vi "Login.vi"(8 "error in (no error)":errorcluster, 11 "UI in":refnum<class "UI.lvclass">) -> (0 "error out":errorcluster, 3 "UI out":refnum<class "UI.lvclass">)   [LabVIEW 2018]
uses:
  User Interface/UI.lvclass
  controls/DataIn.ctl
  MatchDataClasses/MatchData/MatchData.lvclass
  controls/Tabuleiro.ctl
  controls/Table.ctl
  User Interface/UI.lvclass/UI.ctl
  controls/LoginStatus.ctl
  User Interface/getUIData.vi
  User Interface/setUIData.vi
  User Interface/setEmbeddedVI.vi
  <vilib>/Utility/file.llb/Read Delimited Spreadsheet (string).vi
  <vilib>/Utility/file.llb/Write Delimited Spreadsheet (string).vi
panel:
  out "DataOut":T1={"Quem Joga"="", "Tabuleiro"={"(0,0)"="", "(1,0)"="", "(0,1)"="", "(1,1)"="", "(2,0)"="", "(1,2)"="", "(2,2)"="", "(0,2)"="", "(2,1) "=""}, "GameOption"=enum."Multiplayer local", "Turno"=FALSE, "Player"="", "Player 1"="", "Player 2"="", "Dificuldade"=enum."Easy", "Table"=[], "Row"=0, "Aceitar Convite"=FALSE, "Inviter line"=0, "diretório"=path "", "Logout - panel close"=FALSE, "StartGame"=FALSE, "MatchData.lvclass"=refnum, "GameMode"=enum."Single Easy", "Level State"=FALSE}
  out "Table":string[][](table)
  in  "logout":bool
  in  "Login":bool
  in  "User Name":string
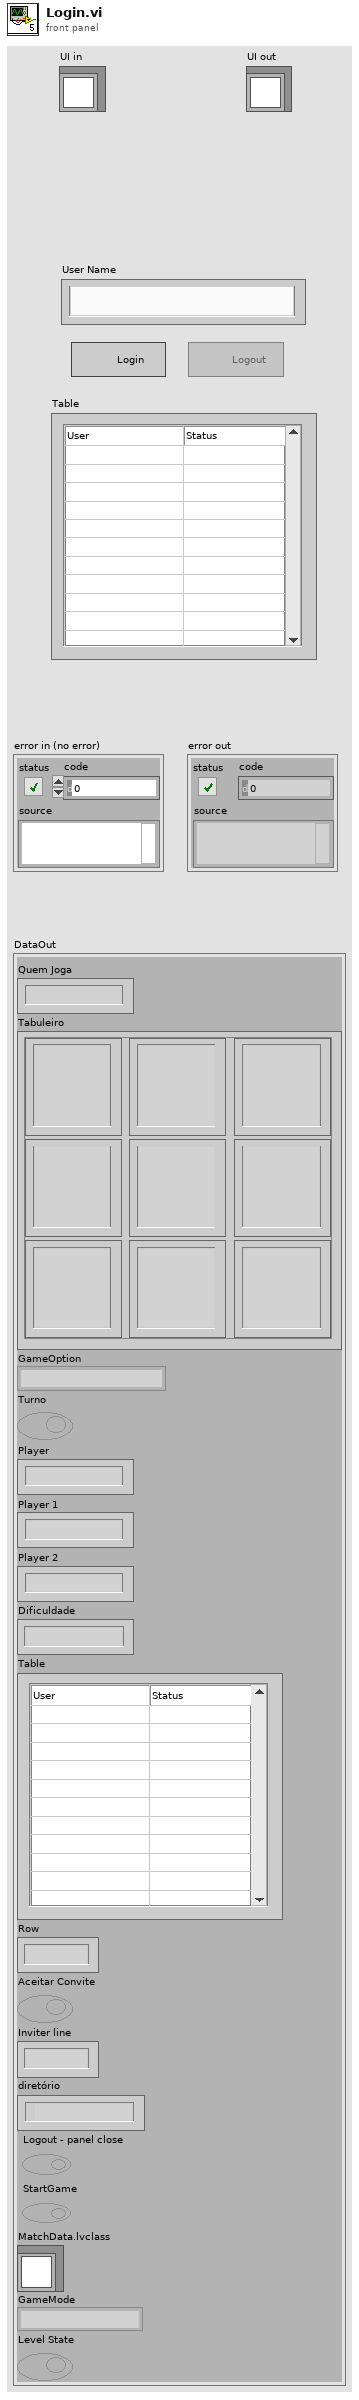
[diagram p1: front panel]
types:
  T1 = typedef "DataIn.ctl" = cluster{"Quem Joga":string, "Tabuleiro":T2, "GameOption":enum16{"Single Player", "Multiplayer local", "Multiplayer remoto", "Wait for Event", "Initialize", "Stop"}, "Turno":bool, "Player":string, "Player 1":string, "Player 2":string, "Dificuldade":enum16{"Easy", "Medium", "Hard"}, "Table":T3, "Row":u32, "Aceitar Convite":bool, "Inviter line":u32, "diretório":path, "Logout - panel close":bool, "StartGame":bool, "MatchData.lvclass":refnum<class "MatchData.lvclass">, "GameMode":enum16{"Single Easy", "Single Medium", "Single Hard", "Local", "Remote"}, "Level State":bool}
  T2 = typedef "Tabuleiro.ctl" = cluster{"(0,0)":string, "(1,0)":string, "(0,1)":string, "(1,1)":string, "(2,0)":string, "(1,2)":string, "(2,2)":string, "(0,2)":string, "(2,1) ":string}
  T3 = typedef "Table.ctl" = string[][]
  T4 = enum8{"Enabled", "Disabled", "Disabled and Grayed Out"}
  T5 = typedef "LoginStatus.ctl" = enum16{"File - Login", "File - Logout", "File - TableRefresh"}
  T6 = typedef "LVRowAndColumnTypeDef.ctl" = cluster{"Row":i32, "Column":i32}
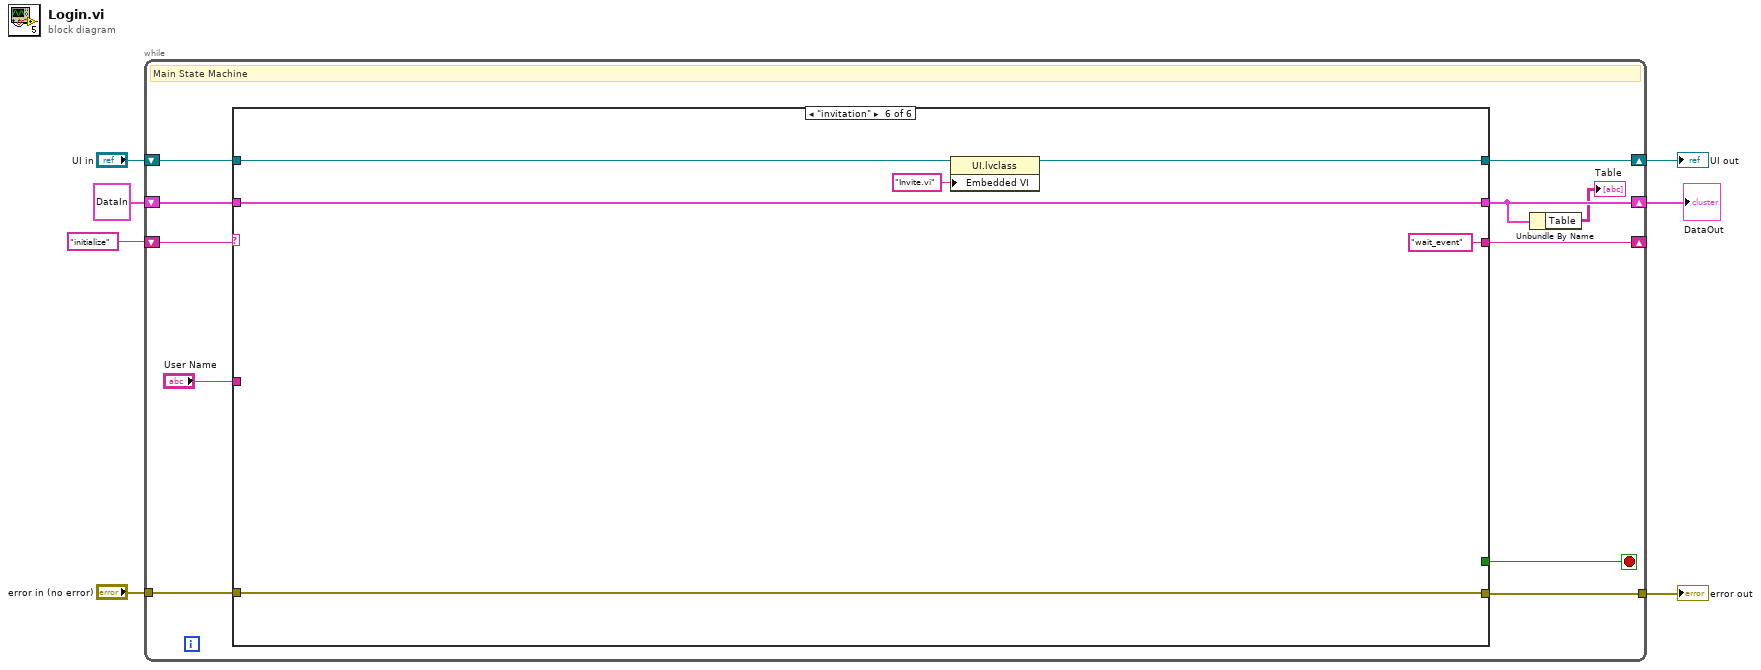
[diagram p0: block diagram]
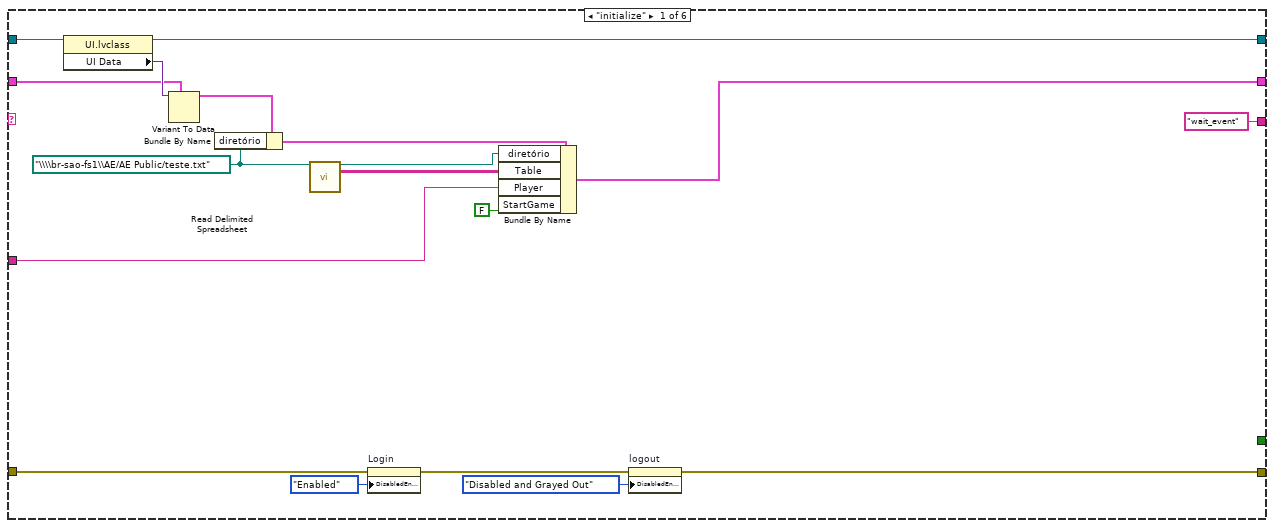
[diagram p2: hidden frame]
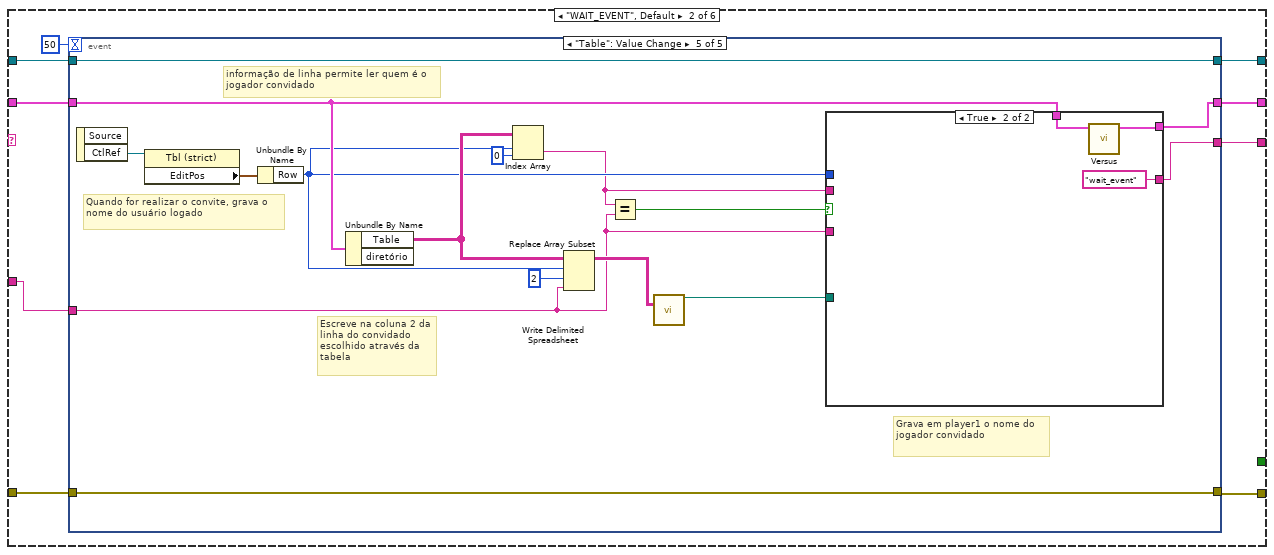
[diagram p3: hidden frame]
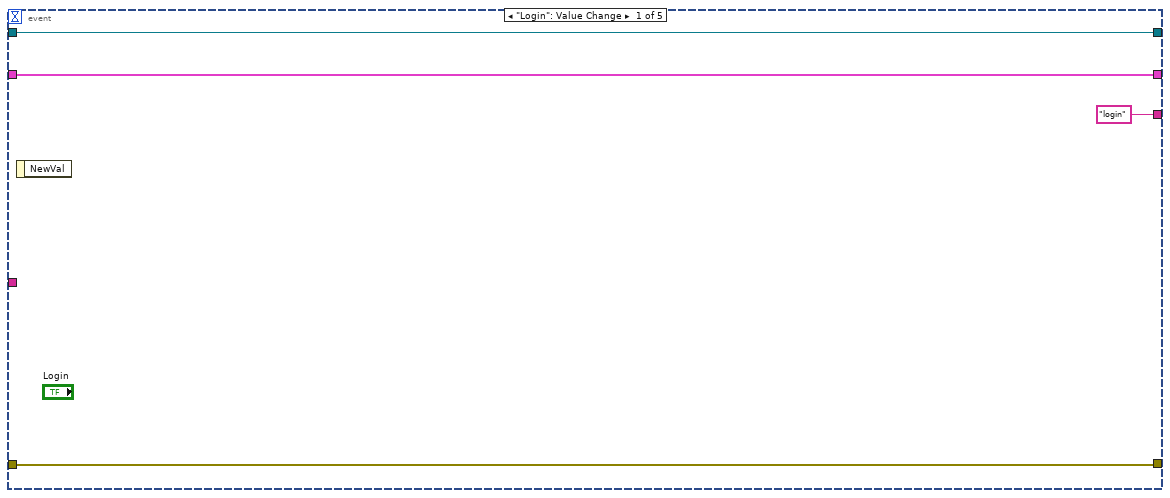
[diagram p4: hidden frame]
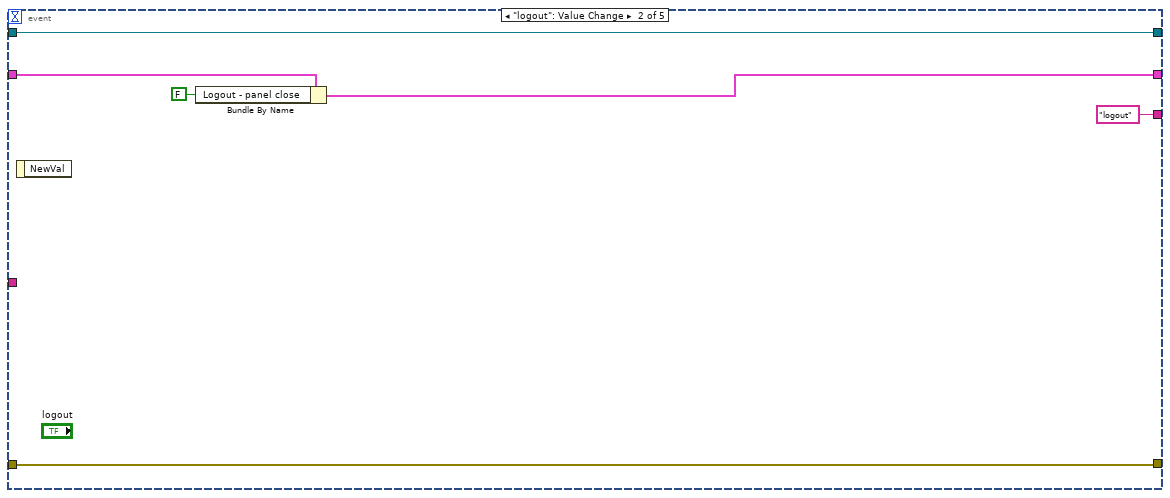
[diagram p5: hidden frame]
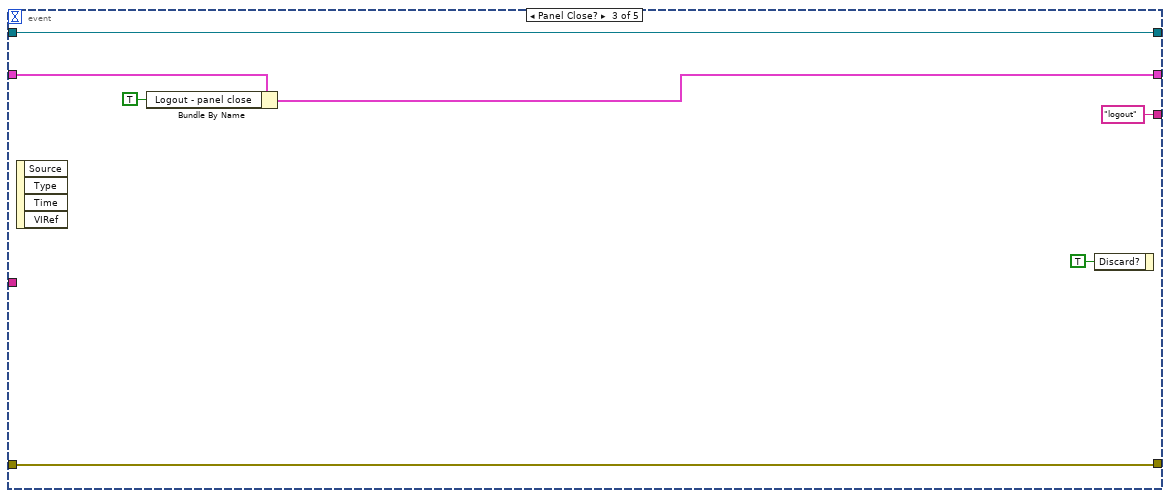
[diagram p6: hidden frame]
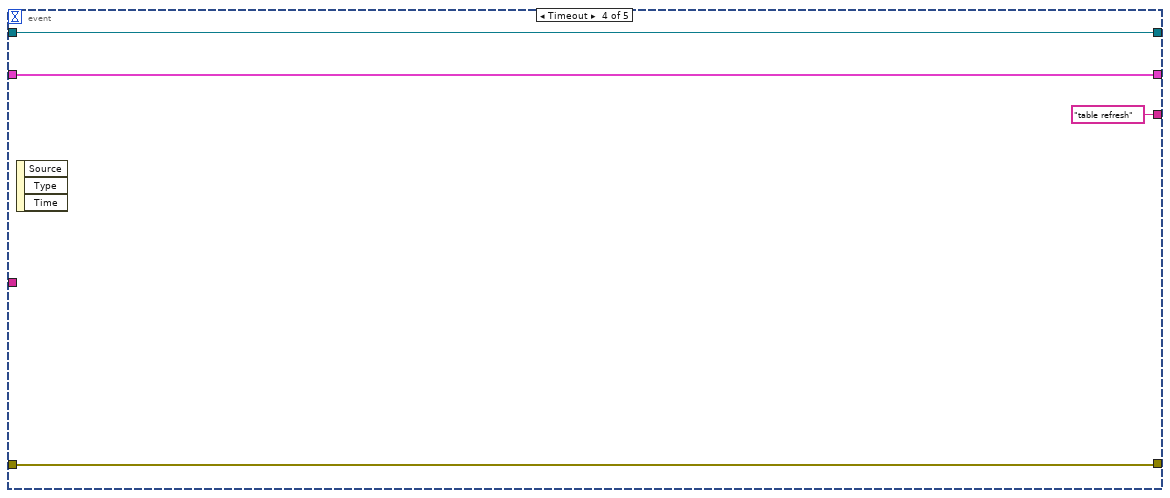
[diagram p7: hidden frame]
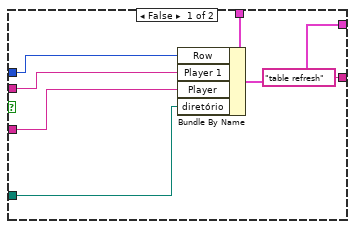
[diagram p8: hidden frame]
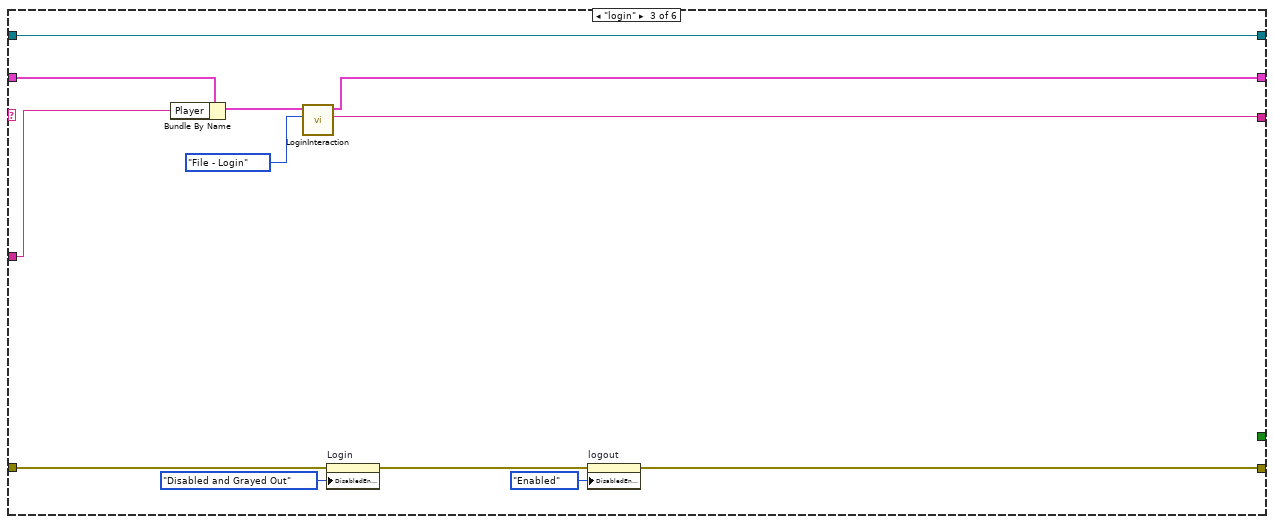
[diagram p9: hidden frame]
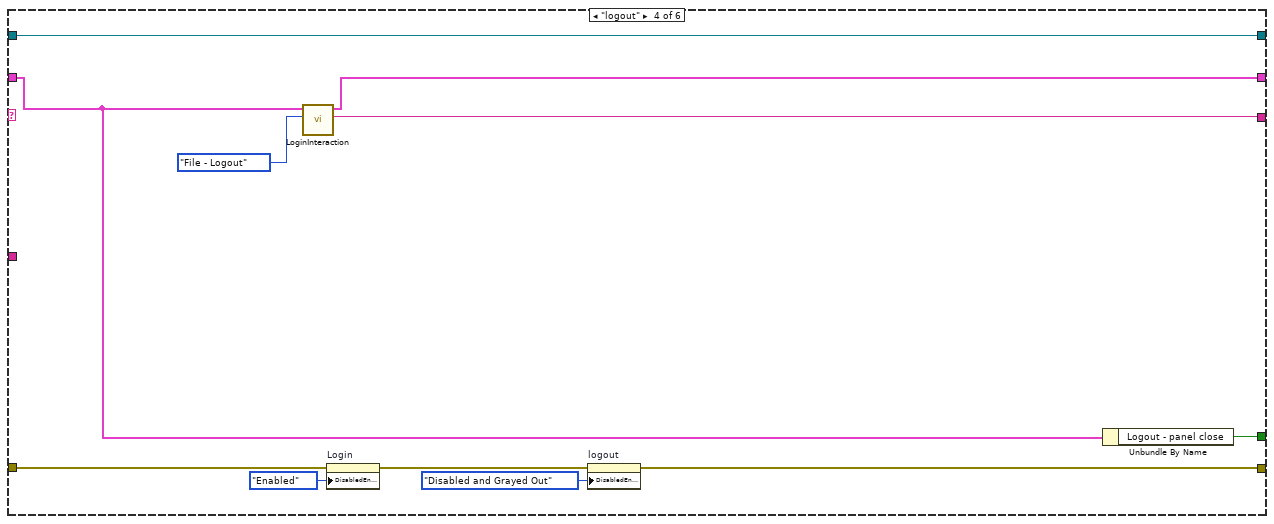
[diagram p10: hidden frame]
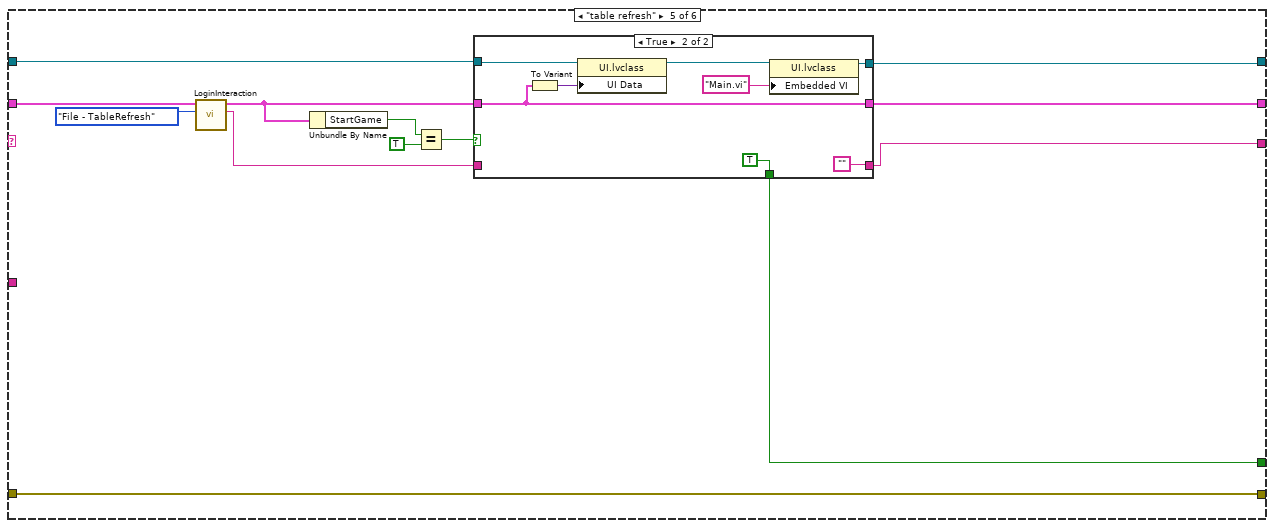
[diagram p11: hidden frame]
diagram:
  n1 = while {
    shift-right: [w17] -> w6
    shift-left: "UI in" -> [w18]
    tunnel: [w16] -> w4
    tunnel: "error in (no error)" -> [w15]
    shift-right: [w14] -> _
    shift-left: "initialize" -> [w12]
    shift-right: [w9] -> w1
    shift-left: T1 {"Quem Joga"="", "Tabuleiro"={"(0,0)"="", "(1,0)"="", "(0,1)"="", "(1,1)"="", "(2,0)"="", "(1,2)"="", "(2,2)"="", "(0,2)"="", "(2,1) "=""}, "GameOption"=enum."Multiplayer local", "Turno"=FALSE, "Player"="", "Player 1"="", "Player 2"="", "Dificuldade"=enum."Easy", "Table"=[], "Row"=0, "Aceitar Convite"=FALSE, "Inviter line"=0, "diretório"=path "", "Logout - panel close"=FALSE, "StartGame"=FALSE, "MatchData.lvclass"=refnum, "GameMode"=enum."Single Easy", "Level State"=FALSE} ("DataIn") -> [w11]
    stop <- w13 stop-if-true
    # "Main State Machine"
    n2 = case shown="\"invitation\"" w12 {
      tunnel: w18 -> [w30 w45 w104 w115 w120 w143]
      tunnel: [w29 w44 w104 w115 w119 w142] -> w17
      tunnel: [w34 w41 w93 w107 w128 w145] -> w16
      tunnel: w15 -> [w36 w43 w94 w108 w128 w145]
      tunnel: ["wait_event" w42 w99 w113 w117 "wait_event" ("Next state")] -> w14
      tunnel: [_ _ _ w105 w116 _] -> w13
      tunnel: w11 -> [w27 w39 w103 w106 w127 w144]
      tunnel: [w19 w40 w100 w114 w121 w144] -> w9
      tunnel: "User Name" -> [w22 w37 w102 _ _ _]
      frame "initialize" {
        w26 = path "\\\\br-sao-fs1\\AE/AE Public/teste.txt" ("file path (use dialog)")
        n3 = property class="UI.lvclass"(reference=w30) -> (reference out=w29:refnum<class "UI.lvclass">, "UI Data"=w28:variant)  [unwired: 1 in, 1 out]
        n4 = Variant To Data(type=w27, Variant=w28) -> (data=w25:T1)  [unwired: 1 in, 1 out]
        n5 = Bundle By Name(cluster=w25, "diretório"=w26) -> (w24:T1)
        n6 = call-poly <vilib>:"Read Delimited Spreadsheet.vi"("file path (dialog if empty)"=w26) -> ("new file path (Not A Path if cancelled)"=w21:path, "all rows"=w20:string[][])  [unwired: 9 in, 4 out]
        n7 = property on="Login" class="Bool"(error in=w36, "DisabledEnum"=T4."Enabled" ("Disabled")) -> (error out=w35:errorcluster)  [unwired: 1 in, 1 out]
        n8 = Bundle By Name(cluster=w24, "diretório"=w21, "Table"=w20, "Player"=w22, "StartGame"=FALSE) -> (w19:T1)
        n9 = property on="logout" class="Bool"(error in=w35, "DisabledEnum"=T4."Disabled and Grayed Out" ("Disabled")) -> (error out=w34:errorcluster)  [unwired: 1 in, 1 out]
      }
      frame "WAIT_EVENT", Default {
        n10 = event shown="[4] \"Table\": Value Change" {
          selector: _ -> [_ _ _ _ _]
          dyn-events: _ -> [_ _ _ _ _]
          timeout: 50 -> [_ _ _ _ _]
          tunnel: [w48 w54 w62 w66 w82] -> w44
          tunnel: w45 -> [w48 w54 w62 w66 w82]
          tunnel: [w49 w55 w61 w65 w81] -> w41
          tunnel: w43 -> [w49 w55 w61 w65 w81]
          tunnel: ["login" "logout" "logout" "table refresh" w70] -> w42
          tunnel: [w46 w50 w57 w63 w71] -> w40
          tunnel: w39 -> [w46 w52 w58 w63 w72]
          tunnel: w37 -> [_ _ _ _ w68]
          event "Login": Value Change {
            n11 = event-data() -> ()  [unwired: 1 in, 1 out]
          }
          event "logout": Value Change {
            n12 = event-data() -> ()  [unwired: 1 in, 1 out]
            n13 = Bundle By Name(cluster=w52, "Logout - panel close"=FALSE) -> (w50:T1)
          }
          event Panel Close? {
            n14 = event-data() -> ()  [unwired: 1 in, 4 out]
            n15 = Bundle By Name(cluster=w58, "Logout - panel close"=TRUE) -> (w57:T1)
            n16 = event-data("Discard?"=TRUE) -> ()  [unwired: 1 in, 1 out]
          }
          event Timeout {
            n17 = event-data() -> ()  [unwired: 1 in, 3 out]
          }
          event "Table": Value Change {
            # "Grava em player1 o nome do  jogador convidado"
            # "Escreve na coluna 2 da linha do convidado escolhido através da tabela"
            # "informação de linha permite ler quem é o jogador convidado"
            # "Quando for realizar o convite, grava o nome do usuário logado"
            n18 = event-data() -> ("CtlRef"=w80:refnum<vi>)  [unwired: 1 in, 1 out]
            n19 = property class="Tbl (strict)"(reference=w80) -> ("EditPos"=w79:T6)  [unwired: 1 in, 2 out]
            n20 = Unbundle By Name(w79) -> ("Row"=w69:i32)
            n21 = Unbundle By Name(w72) -> ("Table"=w76:T3)  [unwired: 1 out]
            n22 = Index Array(array=w76, index (row)=w69, index (col)=0 ("disabled index (col)")) -> (element=w67:string)
            n23 = Replace Array Subset(array=w76, new element=w68, index (row)=w69, index (col)=2 ("disabled index (col)")) -> (w75:T3)
            n24 = Equal?(x=w67, y=w68) -> (x = y?=w74:bool)
            n25 = call-poly <vilib>:"Write Delimited Spreadsheet.vi"("2D data"=w75) -> ("new file path (Not A Path if cancelled)"=w73:path)  [unwired: 13 in, 1 out]
            n26 = case shown="True" w74 {
              tunnel: w73 -> [w83 _]
              tunnel: w72 -> [w89 w91]
              tunnel: [w88 w90] -> w71
              tunnel: ["table refresh" "wait_event"] -> w70
              tunnel: w69 -> [w86 _]
              tunnel: w68 -> [w85 _]
              tunnel: w67 -> [w84 _]
              frame False {
                n27 = Bundle By Name(cluster=w89, "Row"=w86, "Player 1"=w84, "Player"=w85, "diretório"=w83) -> (w88:T1)
              }
              frame True {
                n28 = call "Versus.vi"("DataIn"=w91) -> ("DataOut"=w90:T1)  [unwired: 10 in]
              }
            }
          }
        }
      }
      frame "login" {
        n29 = Bundle By Name(cluster=w103, "Player"=w102) -> (w101:T1)
        n30 = call "LoginInteraction.vi"("LoginStatus"=LoginStatus."File - Login", "DataIn"=w101) -> ("Next state"=w99:string, "DataOut"=w100:T1)  [unwired: 8 in]
        n31 = property on="Login" class="Bool"(error in=w94, "DisabledEnum"=T4."Disabled and Grayed Out" ("Disabled")) -> (error out=w97:errorcluster)  [unwired: 1 in, 1 out]
        n32 = property on="logout" class="Bool"(error in=w97, "DisabledEnum"=T4."Enabled" ("Disabled")) -> (error out=w93:errorcluster)  [unwired: 1 in, 1 out]
      }
      frame "logout" {
        n33 = call "LoginInteraction.vi"("LoginStatus"=LoginStatus."File - Logout", "DataIn"=w106) -> ("Next state"=w113:string, "DataOut"=w114:T1)  [unwired: 8 in]
        n34 = property on="Login" class="Bool"(error in=w108, "DisabledEnum"=T4."Enabled" ("Disabled")) -> (error out=w111:errorcluster)  [unwired: 1 in, 1 out]
        n35 = property on="logout" class="Bool"(error in=w111, "DisabledEnum"=T4."Disabled and Grayed Out" ("Disabled")) -> (error out=w107:errorcluster)  [unwired: 1 in, 1 out]
        n36 = Unbundle By Name(w106) -> ("Logout - panel close"=w105:bool)
      }
      frame "table refresh" {
        n37 = call "LoginInteraction.vi"("LoginStatus"=LoginStatus."File - TableRefresh", "DataIn"=w127) -> ("Next state"=w118:string, "DataOut"=w122:T1)  [unwired: 8 in]
        n38 = Unbundle By Name(w122) -> ("StartGame"=w125:bool)
        n39 = Equal?(x=w125, y=TRUE) -> (x = y?=w123:bool)
        n40 = case shown="True" w123 {
          tunnel: [w131 w134] -> w121
          tunnel: w122 -> [w131 w134]
          tunnel: w120 -> [w130 w138]
          tunnel: [w130 w136] -> w119
          tunnel: w118 -> [w129 _]
          tunnel: [w129 ""] -> w117
          tunnel: [_ TRUE] -> w116
          frame False {
          }
          frame True {
            n41 = To Variant(anything=w134) -> (Variant=w139:variant)
            n42 = property class="UI.lvclass"(reference=w138, "UI Data"=w139) -> (reference out=w137:refnum<class "UI.lvclass">)  [unwired: 1 in, 1 out]
            n43 = property class="UI.lvclass"(reference=w137, "Embedded VI"="Main.vi") -> (reference out=w136:refnum<class "UI.lvclass">)  [unwired: 1 in, 1 out]
          }
        }
      }
      frame "invitation" {
        n44 = property class="UI.lvclass"(reference=w143, "Embedded VI"="Invite.vi") -> (reference out=w142:refnum<class "UI.lvclass">)  [unwired: 1 in, 1 out]
      }
    }
    n45 = Unbundle By Name(w9) -> ("Table"=→"Table":T3)
  }
  "UI out" <- w6
  "error out" <- w4
  "DataOut" <- w1
